vi "stop_action.vi"(0 "HGF_ImaqFg":refnum<class "HGF_ImaqFg.lvclass">, 5 "error in (no error)":errorcluster) -> (14 "dup HGF_ImaqFg":refnum<class "HGF_ImaqFg.lvclass">, 19 "error out":errorcluster)   [LabVIEW 2014, in "HGF_IMAQ.lvlib" / "HGF_ImaqFg.lvclass"]
doc: "Stops an acquisition previously started with IMAQdx Start Acquisition.vi."
uses:
  HGF_ImaqFg.lvclass
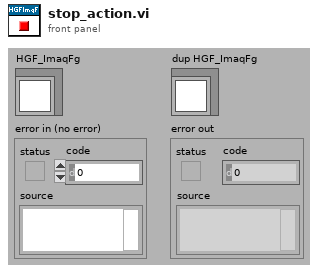
[diagram p1: front panel]
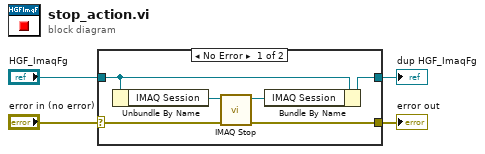
[diagram p0: block diagram]
diagram:
  n1 = case shown="No Error" "error in (no error)" {
    selector: "error in (no error)" -> [w5 w11]
    tunnel: "HGF_ImaqFg" -> [w9 w12]
    tunnel: [w7 w12] -> w1
    tunnel: [w6 w11] -> w2
    frame No Error {
      n2 = Unbundle By Name(w9) -> ("IMAQ Session"=w10:refnum<k11>)
      n3 = call <vilib>:"IMAQ Stop.vi"("error in (no error)"=w5, "IMAQ Session In"=w10) -> ("error out"=w6:errorcluster, "IMAQ Session Out"=w8:refnum<k11>)  [unwired: 8 out]
      n4 = Bundle By Name(cluster=w9, "IMAQ Session"=w8) -> (w7:refnum<class "HGF_ImaqFg.lvclass">)
    }
    frame Error {
    }
  }
  "error out" <- w2
  "dup HGF_ImaqFg" <- w1
